vi "Main 2.0.vi"() -> ()   [LabVIEW 2022 SP3]
uses:
  <vilib>/MakerHub/LINX/Public/Utilities/Open Serial.vi
  <vilib>/MakerHub/LINX/Public/Sensors/Motion/Servo/Servo Open One Channel.vi
  Global 2 Horizontal.vi
  Global 3 Vertical.vi
  Global 4 Gripper.vi
  <vilib>/MakerHub/LINX/Public/Sensors/Motion/Servo/Servo Set Pulse Width One Channel.vi
  <vilib>/MakerHub/LINX/Public/Sensors/Motion/Servo/Servo Close One Channel.vi
  Global 1 Base.vi
  <vilib>/MakerHub/LINX/LMH-LINX.lvlib
  <vilib>/MakerHub/LINX/Public/Sensors/Motion/Servo/Servo.lvlib
panel:
  in  "Slide 4":i32(slide) scale=0.0..140.0
  in  "Slide 3":i32(slide) scale=90.0..160.0
  in  "Slide 2":i32(slide) scale=50.0..160.0
  in  "Slide":i32(slide) scale=-70.0..250.0
  out "Square":dynamicdata(graph)
  in  "stop":bool
  in  "Arm":bool
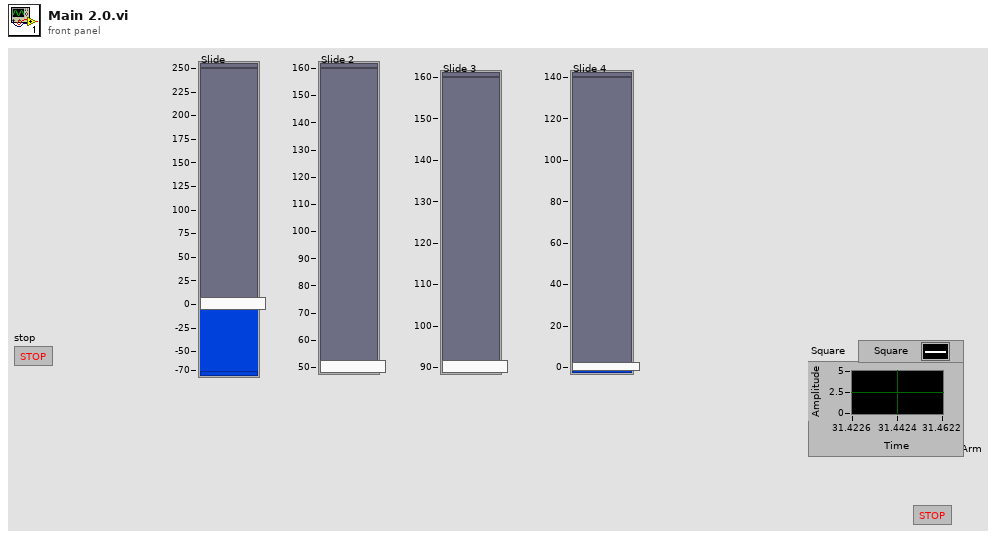
[diagram p1: front panel]
types:
  T1 = typedef "LMH-LINX.lvlib/LINX Ref.ctl" = cluster{"IO":T2, "Interface":T3, "LINX Device Config":T4}
  T2 = typedef "LMH-LINX.lvlib/Platform.ctl" = enum16{"Remote", "Local"}
  T3 = typedef "LMH-LINX.lvlib/Interface.ctl" = enum16{"Serial", "TCP"}
  T4 = typedef "LMH-LINX.lvlib/Device.lvlib/LINX Device Config.ctl" = cluster{"Interface":T3, "COM Port":refnum<visa-resource-name>, "TCP Configuration":T5, "Device Family":u8, "Device ID":u8, "Device Name":string, "TCP Ref":refnum<k5>, "Channels":T6}
  T5 = typedef "LMH-LINX.lvlib/Device.lvlib/TCP Config.ctl" = cluster{"IP Address":string, "Port":u16}
  T6 = typedef "LMH-LINX.lvlib/Channels.ctl" = cluster{"DI":u8[], "DO":u8[], "AI":u8[], "AO":u8[], "PWM":u8[], "QE":u8[], "UART":u8[], "I2C 2":u8[], "SPI":u8[], "CAN":u8[], "Servo":u8[], "AI Ref (V)":dbl, "AI Resolution (Bits)":u8, "AO Ref (V)":dbl, "AO Resolution (Bits)":u8}
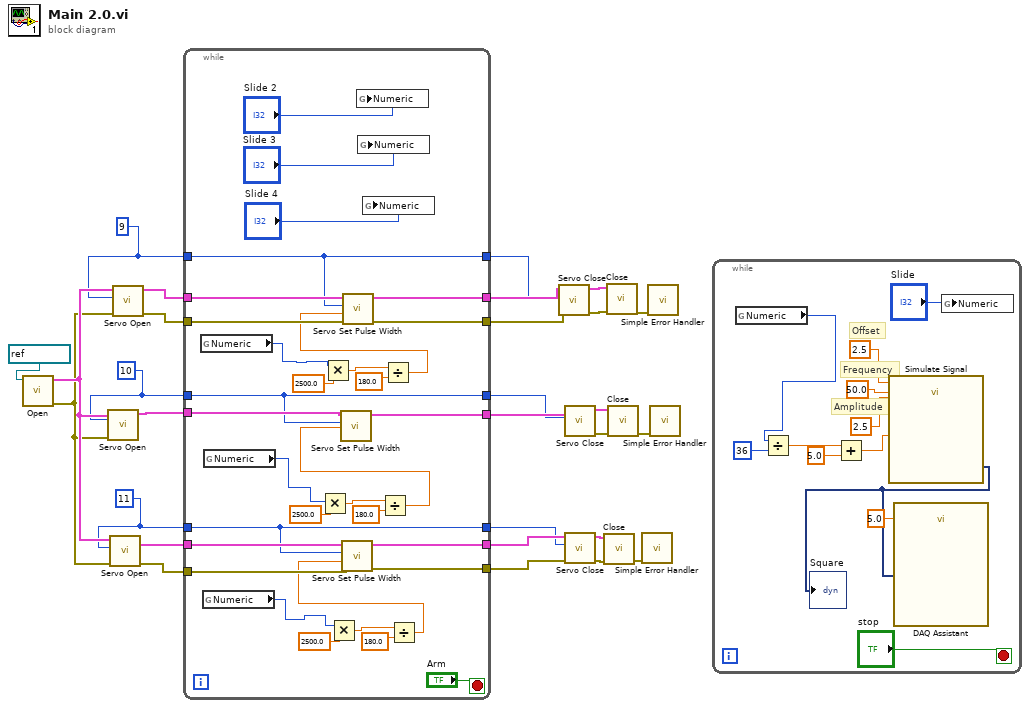
[diagram p0: block diagram]
diagram:
  w6 = 11
  w4 = 10
  w1 = 9
  n1 = call-poly <vilib>:"Open.vi"("Serial Port"=refnum<visa-resource-name> "COM6") -> ("Error Out"=w7:errorcluster, "LINX Resource"=w8:T1)  [unwired: 8 in, 1 out]
  n2 = call-poly <vilib>:"Servo Open.vi"("Error In"=w7, "Servo Channel"=w4, "LINX Resource"=w8) -> ("LINX Resource"=w14:T1)  [unwired: 7 in, 1 out]
  n3 = call-poly <vilib>:"Servo Open.vi"("Error In"=w7, "Servo Channel"=w6, "LINX Resource"=w8) -> ("Error Out"=w10:errorcluster, "LINX Resource"=w11:T1)  [unwired: 7 in]
  n4 = call-poly <vilib>:"Servo Open.vi"("Error In"=w7, "Servo Channel"=w1, "LINX Resource"=w8) -> ("Error Out"=w25:errorcluster, "LINX Resource"=w27:T1)  [unwired: 7 in]
  n5 = while {
    tunnel: w27 -> [w59]
    tunnel: [w58] -> w26
    tunnel: w25 -> [w57]
    tunnel: [w56] -> w24
    tunnel: w1 -> [w47]
    tunnel: w14 -> [w55]
    tunnel: [w54] -> w13
    tunnel: [w53] -> w12
    tunnel: w11 -> [w52]
    tunnel: w10 -> [w51]
    tunnel: [w50] -> w9
    tunnel: w6 -> [w49]
    tunnel: [w49] -> w5
    tunnel: w4 -> [w48]
    tunnel: [w48] -> w3
    tunnel: [w47] -> w2
    stop <- "Arm" stop-if-true
    n6 = global read "Global 2 Horizontal.vi" "Numeric"() -> (w32:i32)
    n7 = global read "Global 4 Gripper.vi" "Numeric"() -> (w34:i32)
    n8 = global read "Global 3 Vertical.vi" "Numeric"() -> (w33:i32)
    n9 = Multiply(x=w33, y=2500.0) -> (x*y=w43:dbl)
    n10 = Multiply(x=w32, y=2500.0) -> (x*y=w46:dbl)
    n11 = Multiply(x=w34, y=2500.0) -> (x*y=w40:dbl)
    n12 = global write "Global 2 Horizontal.vi" "Numeric"("Slide 2") -> ()
    n13 = global write "Global 3 Vertical.vi" "Numeric"("Slide 3") -> ()
    n14 = global write "Global 4 Gripper.vi" "Numeric"("Slide 4") -> ()
    n15 = Divide(x=w43, y=180.0) -> (x/y=w36:dbl)
    n16 = call-poly <vilib>:"Servo Set Pulse Width.vi"("Pulse Width (uS)"=w36, "Servo Channel"=w48, "LINX Resource"=w55) -> ("LINX Resource"=w54:T1)  [unwired: 7 in, 1 out]
    n17 = Divide(x=w46, y=180.0) -> (x/y=w35:dbl)
    n18 = call-poly <vilib>:"Servo Set Pulse Width.vi"("Error In"=w57, "Pulse Width (uS)"=w35, "Servo Channel"=w47, "LINX Resource"=w59) -> ("Error Out"=w56:errorcluster, "LINX Resource"=w58:T1)  [unwired: 6 in]
    n19 = Divide(x=w40, y=180.0) -> (x/y=w37:dbl)
    n20 = call-poly <vilib>:"Servo Set Pulse Width.vi"("Error In"=w51, "Pulse Width (uS)"=w37, "Servo Channel"=w49, "LINX Resource"=w52) -> ("Error Out"=w50:errorcluster, "LINX Resource"=w53:T1)  [unwired: 6 in]
  }
  n21 = call-poly <vilib>:"Servo Close.vi"("Error In"=w24, "Servo Channel"=w2, "LINX Resource"=w26) -> ("Error Out"=w21:errorcluster, "LINX Resource"=w22:T1)  [unwired: 7 in]
  n22 = call-poly <vilib>:"Servo Close.vi"("Servo Channel"=w3, "LINX Resource"=w13) -> ("Error Out"=w18:errorcluster, "LINX Resource"=w19:T1)  [unwired: 8 in]
  n23 = call-poly <vilib>:"Servo Close.vi"("Error In"=w9, "Servo Channel"=w5, "LINX Resource"=w12) -> ("Error Out"=w15:errorcluster, "LINX Resource"=w16:T1)  [unwired: 7 in]
  n24 = call <vilib>:"Close.vi"("Error In"=w15, "LINX Resource"=w16) -> ("Error Out"=w17:errorcluster)  [unwired: 9 in]
  n25 = call <vilib>:"Close.vi"("Error In"=w21, "LINX Resource"=w22) -> ("Error Out"=w23:errorcluster)  [unwired: 9 in]
  n26 = call <vilib>:"Close.vi"("Error In"=w18, "LINX Resource"=w19) -> ("Error Out"=w20:errorcluster)  [unwired: 9 in]
  n27 = call <vilib>:"Simple Error Handler.vi"("error in (no error)"=w17) -> ()  [unwired: 4 in, 5 out]
  n28 = call <vilib>:"Simple Error Handler.vi"("error in (no error)"=w23) -> ()  [unwired: 4 in, 5 out]
  n29 = call <vilib>:"Simple Error Handler.vi"("error in (no error)"=w20) -> ()  [unwired: 4 in, 5 out]
  n30 = while {
    stop <- "stop" stop-if-true
    # "Amplitude"
    # "Frequency"
    # "Offset"
    n31 = global read "Global 1 Base.vi" "Numeric"() -> (w62:i32)
    n32 = Divide(x=w62, y=36) -> (x/y=w65:dbl)
    n33 = Add(x=w65, y=5.0) -> (x+y=w66:dbl)
    n34 = call "Simulate Signal"("Offset"=2.5, "Duty Cycle (%)"=w66, "Frequency"=50.0, "Amplitude"=2.5) -> ("Square"=w72:dynamicdata)  [unwired: 10 in, 1 out]
    "Square" <- w72
    n35 = call "DAQ Assistant"("data"=w72, "timeout (s)"=5.0) -> ()  [unwired: 15 in, 3 out]
    n36 = global write "Global 1 Base.vi" "Numeric"("Slide") -> ()
  }
